vi "TDMS2TDMData.vi"(0 "tdms file in":refnum<k34>, 1 "Chunk Size":i64, 5 "group name":string, 9 "channel name":string, 11 "error in (no error)":errorcluster, 12 "Data type":i32, 13 "storage refnum":refnum<k20>) -> (4 "tdms file out":refnum<k34>, 6 "group name out":string, 15 "error out":errorcluster)   [LabVIEW 2017]
doc: "This VI transfers channel data from a TDMS channel to a TDM channel. The data is transfered in chunks of a certain size measured in samples until all the transfer is complete. If the TDMS channel contains a datatype not supported by the TDM storage format, then the data is coerced and the coercion is logged."
uses:
  <vilib>/Platform/storage/lvStorage.llb/_saveUInt8Channel.vi
  <vilib>/Utility/tdmsutil.llb/TDMS2TDMLogDataConversion.vi
  <vilib>/Platform/storage/lvStorage.llb/_saveInt16Channel.vi
  <vilib>/Platform/storage/lvStorage.llb/_saveInt32Channel.vi
  <vilib>/Platform/storage/lvStorage.llb/_saveFloat32Channel.vi
  <vilib>/Platform/storage/lvStorage.llb/_saveFloat64Channel.vi
  <vilib>/Platform/storage/lvStorage.llb/_saveStringChannel.vi
  <vilib>/Platform/storage/lvStorage.llb/_saveDateTimeChannel.vi
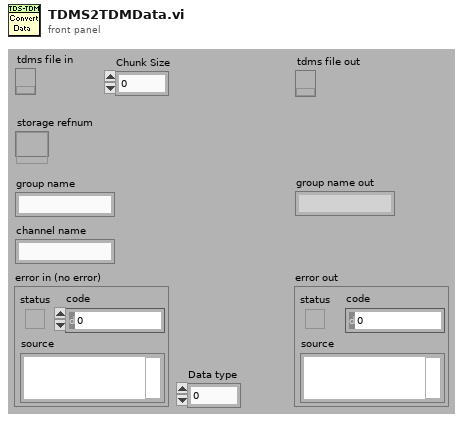
[diagram p1: front panel]
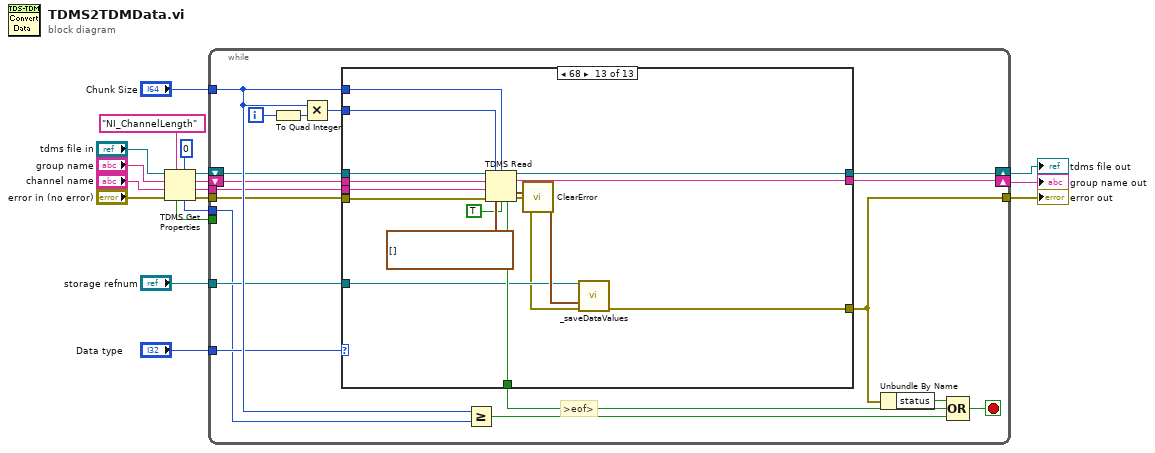
[diagram p0: block diagram]
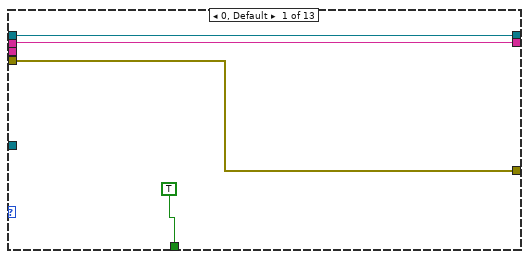
[diagram p2: hidden frame]
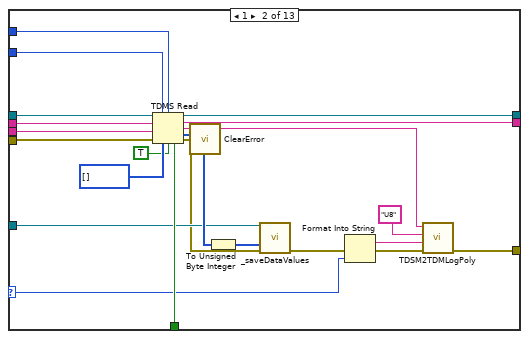
[diagram p3: hidden frame]
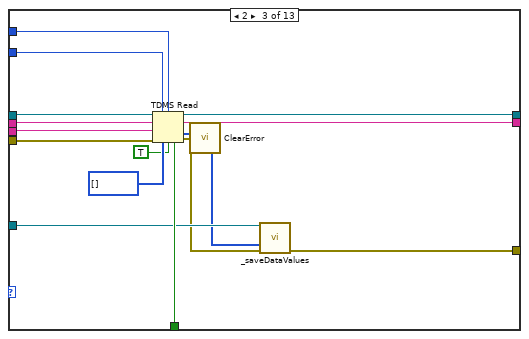
[diagram p4: hidden frame]
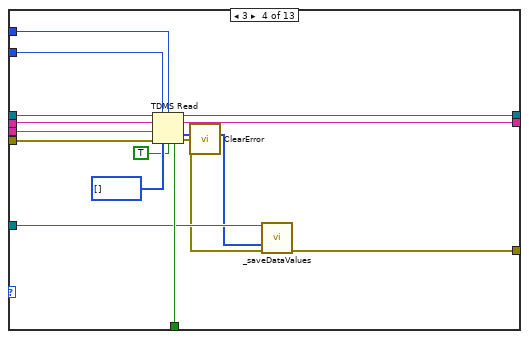
[diagram p5: hidden frame]
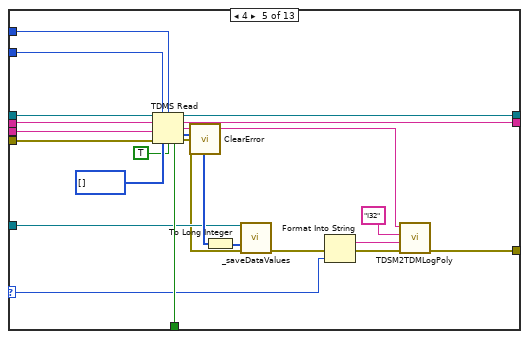
[diagram p6: hidden frame]
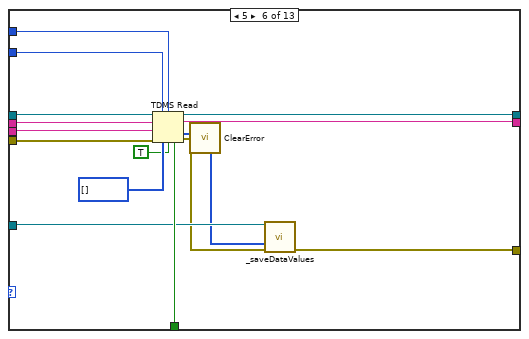
[diagram p7: hidden frame]
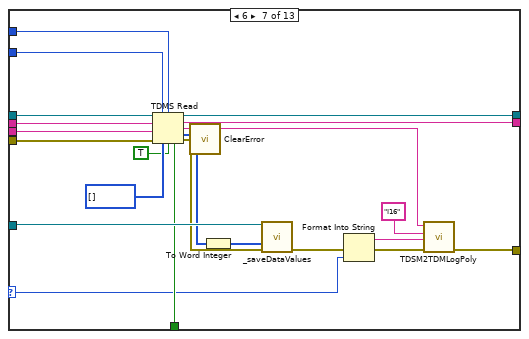
[diagram p8: hidden frame]
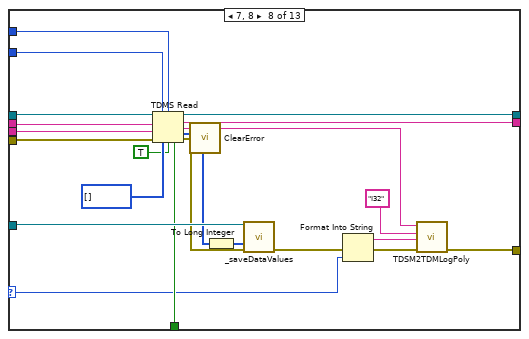
[diagram p9: hidden frame]
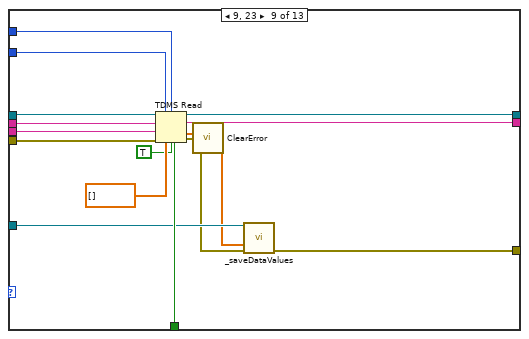
[diagram p10: hidden frame]
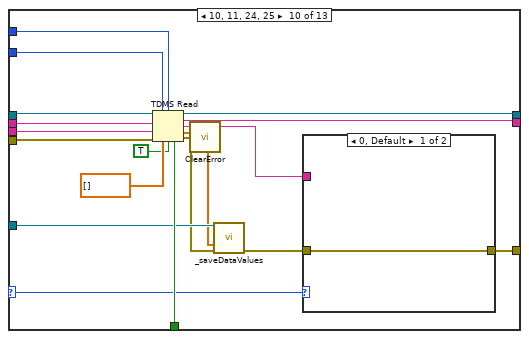
[diagram p11: hidden frame]
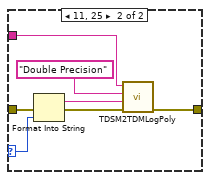
[diagram p12: hidden frame]
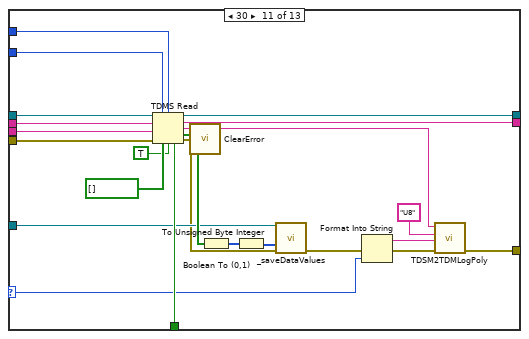
[diagram p13: hidden frame]
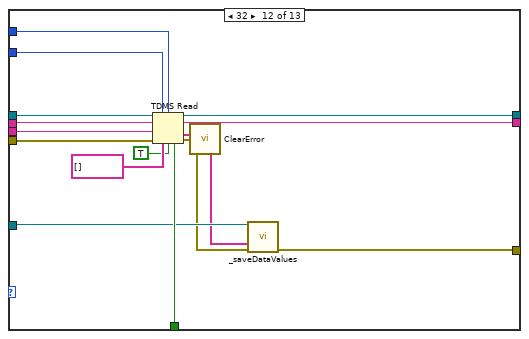
[diagram p14: hidden frame]
diagram:
  n1 = TDMS Get Properties(5:i64 0, 7:"NI_ChannelLength" ("property name"), 8:"error in (no error)", 9:"channel name", 10:"group name", 11:"tdms file in") -> (0:w5:errorcluster, 1:w6:string, 2:w7:string, 3:w8:refnum<k34>, 4:w3:i64, 6:w2:bool)
  n2 = while {
    tunnel: "storage refnum" -> [w34]
    tunnel: w6 -> [w31]
    tunnel: w5 -> [w30]
    shift-right: [w29] -> w15
    shift-left: w8 -> [w33]
    shift-right: [w28] -> w16
    shift-left: w7 -> [w32]
    tunnel: "Chunk Size" -> [w36]
    tunnel: [w35] -> w18
    tunnel: "Data type" -> [w24]
    tunnel: w3 -> [w21]
    tunnel: w2 -> [_]
    i -> [w27]
    stop <- w19 stop-if-true
    # ">eof>"
    n3 = To Quad Integer(1:w27) -> (0:w26:i64)
    n4 = Multiply(x=w36, y=w26) -> (x*y=w25:i64)
    n5 = case shown="68" w24 {
      selector: w24 -> [_ w46 _ _ w103 _ w142 w162 _ w202 w229 _ _]
      tunnel: w34 -> [_ w52 w68 w84 w107 w124 w157 w180 w185 w205 w236 w254 w269]
      tunnel: w33 -> [w40 w63 w79 w95 w118 w134 w156 w179 w196 w215 w247 w263 w279]
      tunnel: w32 -> [w39 w62 w78 w93 w117 w131 w154 w177 w194 w213 w244 w261 w278]
      tunnel: w31 -> [_ w61 w77 w92 w116 w130 w153 w176 w193 w212 w243 w256 w277]
      tunnel: w30 -> [w37 w60 w74 w91 w115 w128 w151 w178 w195 w211 w238 w260 w271]
      tunnel: [w40 w57 w76 w94 w113 w133 w155 w174 w192 w214 w246 w262 w276] -> w29
      tunnel: [w39 w56 w75 w89 w112 w129 w152 w173 w191 w206 w245 w255 w275] -> w28
      tunnel: w25 -> [_ w54 w71 w86 w110 w125 w148 w171 w188 w209 w240 w257 w273]
      tunnel: w36 -> [_ w55 w70 w87 w111 w126 w149 w172 w189 w210 w241 w258 w274]
      tunnel: [w37 w49 w69 w85 w101 w123 w139 w164 w186 w200 w230 w253 w268] -> w35
      tunnel: [TRUE ("eof") w53 w73 w90 w109 w132 w150 w175 w190 w208 w242 w259 w272] -> w22
      frame 0, Default {
      }
      frame 1 {
        n6 = TDMS Read(0:w63, 1:w54, 2:w55, 5:w62, 7:w61, 11:w60, 12:i8[] [], 13:TRUE ("return channels in file order? (F)")) -> (4:w57:refnum<k34>, 6:w56:string, 8:w43:string, 10:w59:i8[], 14:w53:bool, 15:w42:errorcluster)
        n7 = call <vilib>:"ClearError.vi"("error in (no error)"=w42) -> ("error out"=w50:errorcluster)
        n8 = To Unsigned Byte Integer(number=w59) -> (unsigned 8bit integer=w51:u8[])
        n9 = call-poly <vilib>:"_saveDataValues.vi"("Data object in"=w52, "Values"=w51, "error in (no error)"=w50) -> ("error out"=w48:errorcluster)  [unwired: 10 in, 2 out]
        n10 = Format Into String(error in=w48, w46) -> (resulting string=w45:string, error out=w47:errorcluster)  [unwired: 2 in]
        n11 = call-poly <vilib>:"TDSM2TDMLogPoly.vi"("error in (no error)"=w47, "Original Datatype"=w45, "New Datatype"="U8", "Channel Name"=w43) -> ("error out"=w49:errorcluster)  [unwired: 7 in]
      }
      frame 2 {
        n12 = TDMS Read(0:w79, 1:w71, 2:w70, 5:w78, 7:w77, 11:w74, 12:i16[] [], 13:TRUE ("return channels in file order? (F)")) -> (4:w76:refnum<k34>, 6:w75:string, 10:w67:i16[], 14:w73:bool, 15:w65:errorcluster)  [unwired: 1 out]
        n13 = call <vilib>:"ClearError.vi"("error in (no error)"=w65) -> ("error out"=w66:errorcluster)
        n14 = call-poly <vilib>:"_saveDataValues.vi"("Data object in"=w68, "Values"=w67, "error in (no error)"=w66) -> ("error out"=w69:errorcluster)  [unwired: 10 in, 2 out]
      }
      frame 3 {
        n15 = TDMS Read(0:w95, 1:w86, 2:w87, 5:w93, 7:w92, 11:w91, 12:i32[] [], 13:TRUE ("return channels in file order? (F)")) -> (4:w94:refnum<k34>, 6:w89:string, 10:w83:i32[], 14:w90:bool, 15:w81:errorcluster)  [unwired: 1 out]
        n16 = call <vilib>:"ClearError.vi"("error in (no error)"=w81) -> ("error out"=w82:errorcluster)
        n17 = call-poly <vilib>:"_saveDataValues.vi"("Data object in"=w84, "Values"=w83, "error in (no error)"=w82) -> ("error out"=w85:errorcluster)  [unwired: 10 in, 2 out]
      }
      frame 4 {
        n18 = TDMS Read(0:w118, 1:w110, 2:w111, 5:w117, 7:w116, 11:w115, 12:i64[] [], 13:TRUE ("return channels in file order? (F)")) -> (4:w113:refnum<k34>, 6:w112:string, 8:w98:string, 10:w108:i64[], 14:w109:bool, 15:w97:errorcluster)
        n19 = call <vilib>:"ClearError.vi"("error in (no error)"=w97) -> ("error out"=w105:errorcluster)
        n20 = To Long Integer(number=w108) -> (32bit integer=w106:i32[])
        n21 = call-poly <vilib>:"_saveDataValues.vi"("Data object in"=w107, "Values"=w106, "error in (no error)"=w105) -> ("error out"=w104:errorcluster)  [unwired: 10 in, 2 out]
        n22 = Format Into String(error in=w104, w103) -> (resulting string=w100:string, error out=w102:errorcluster)  [unwired: 2 in]
        n23 = call-poly <vilib>:"TDSM2TDMLogPoly.vi"("error in (no error)"=w102, "Original Datatype"=w100, "New Datatype"="I32", "Channel Name"=w98) -> ("error out"=w101:errorcluster)  [unwired: 7 in]
      }
      frame 5 {
        n24 = TDMS Read(0:w134, 1:w125, 2:w126, 5:w131, 7:w130, 11:w128, 12:u8[] [], 13:TRUE ("return channels in file order? (F)")) -> (4:w133:refnum<k34>, 6:w129:string, 10:w122:u8[], 14:w132:bool, 15:w120:errorcluster)  [unwired: 1 out]
        n25 = call <vilib>:"ClearError.vi"("error in (no error)"=w120) -> ("error out"=w121:errorcluster)
        n26 = call-poly <vilib>:"_saveDataValues.vi"("Data object in"=w124, "Values"=w122, "error in (no error)"=w121) -> ("error out"=w123:errorcluster)  [unwired: 10 in, 2 out]
      }
      frame 6 {
        n27 = TDMS Read(0:w156, 1:w148, 2:w149, 5:w154, 7:w153, 11:w151, 12:u16[] [], 13:TRUE ("return channels in file order? (F)")) -> (4:w155:refnum<k34>, 6:w152:string, 8:w137:string, 10:w146:u16[], 14:w150:bool, 15:w136:errorcluster)
        n28 = call <vilib>:"ClearError.vi"("error in (no error)"=w136) -> ("error out"=w144:errorcluster)
        n29 = To Word Integer(number=w146) -> (16bit integer=w145:i16[])
        n30 = call-poly <vilib>:"_saveDataValues.vi"("Data object in"=w157, "Values"=w145, "error in (no error)"=w144) -> ("error out"=w143:errorcluster)  [unwired: 10 in, 2 out]
        n31 = Format Into String(error in=w143, w142) -> (resulting string=w140:string, error out=w141:errorcluster)  [unwired: 2 in]
        n32 = call-poly <vilib>:"TDSM2TDMLogPoly.vi"("error in (no error)"=w141, "Original Datatype"=w140, "New Datatype"="I16", "Channel Name"=w137) -> ("error out"=w139:errorcluster)  [unwired: 7 in]
      }
      frame 7, 8 {
        n33 = TDMS Read(0:w179, 1:w171, 2:w172, 5:w177, 7:w176, 11:w178, 12:u32[] [], 13:TRUE ("return channels in file order? (F)")) -> (4:w174:refnum<k34>, 6:w173:string, 8:w160:string, 10:w169:u32[], 14:w175:bool, 15:w159:errorcluster)
        n34 = call <vilib>:"ClearError.vi"("error in (no error)"=w159) -> ("error out"=w167:errorcluster)
        n35 = To Long Integer(number=w169) -> (32bit integer=w168:i32[])
        n36 = call-poly <vilib>:"_saveDataValues.vi"("Data object in"=w180, "Values"=w168, "error in (no error)"=w167) -> ("error out"=w166:errorcluster)  [unwired: 10 in, 2 out]
        n37 = Format Into String(error in=w166, w162) -> (resulting string=w163:string, error out=w165:errorcluster)  [unwired: 2 in]
        n38 = call-poly <vilib>:"TDSM2TDMLogPoly.vi"("error in (no error)"=w165, "Original Datatype"=w163, "New Datatype"="I32", "Channel Name"=w160) -> ("error out"=w164:errorcluster)  [unwired: 7 in]
      }
      frame 9, 23 {
        n39 = TDMS Read(0:w196, 1:w188, 2:w189, 5:w194, 7:w193, 11:w195, 12:sgl[] [], 13:TRUE ("return channels in file order? (F)")) -> (4:w192:refnum<k34>, 6:w191:string, 10:w183:sgl[], 14:w190:bool, 15:w182:errorcluster)  [unwired: 1 out]
        n40 = call <vilib>:"ClearError.vi"("error in (no error)"=w182) -> ("error out"=w184:errorcluster)
        n41 = call-poly <vilib>:"_saveDataValues.vi"("Data object in"=w185, "Values"=w183, "error in (no error)"=w184) -> ("error out"=w186:errorcluster)  [unwired: 10 in, 2 out]
      }
      frame 10, 11, 24, 25 {
        n42 = TDMS Read(0:w215, 1:w209, 2:w210, 5:w213, 7:w212, 11:w211, 12:dbl[] [], 13:TRUE ("return channels in file order? (F)")) -> (4:w214:refnum<k34>, 6:w206:string, 8:w199:string, 10:w204:dbl[], 14:w208:bool, 15:w198:errorcluster)
        n43 = call <vilib>:"ClearError.vi"("error in (no error)"=w198) -> ("error out"=w203:errorcluster)
        n44 = call-poly <vilib>:"_saveDataValues.vi"("Data object in"=w205, "Values"=w204, "error in (no error)"=w203) -> ("error out"=w201:errorcluster)  [unwired: 10 in, 2 out]
        n45 = case shown="0, Default" w202 {
          selector: w202 -> [_ w222]
          tunnel: w201 -> [w216 w223]
          tunnel: [w216 w219] -> w200
          tunnel: w199 -> [_ w217]
          frame 0, Default {
          }
          frame 11, 25 {
            n46 = Format Into String(error in=w223, w222) -> (resulting string=w220:string, error out=w221:errorcluster)  [unwired: 2 in]
            n47 = call-poly <vilib>:"TDSM2TDMLogPoly.vi"("error in (no error)"=w221, "Original Datatype"=w220, "New Datatype"="Double Precision", "Channel Name"=w217) -> ("error out"=w219:errorcluster)  [unwired: 7 in]
          }
        }
      }
      frame 30 {
        n48 = TDMS Read(0:w247, 1:w240, 2:w241, 5:w244, 7:w243, 11:w238, 12:bool[] [], 13:TRUE ("return channels in file order? (F)")) -> (4:w246:refnum<k34>, 6:w245:string, 8:w226:string, 10:w237:bool[], 14:w242:bool, 15:w225:errorcluster)
        n49 = call <vilib>:"ClearError.vi"("error in (no error)"=w225) -> ("error out"=w235:errorcluster)
        n50 = Boolean To (0,1)(Boolean=w237) -> (0, 1=w234:i16[])
        n51 = To Unsigned Byte Integer(number=w234) -> (unsigned 8bit integer=w233:u8[])
        n52 = call-poly <vilib>:"_saveDataValues.vi"("Data object in"=w236, "Values"=w233, "error in (no error)"=w235) -> ("error out"=w232:errorcluster)  [unwired: 10 in, 2 out]
        n53 = Format Into String(error in=w232, w229) -> (resulting string=w228:string, error out=w231:errorcluster)  [unwired: 2 in]
        n54 = call-poly <vilib>:"TDSM2TDMLogPoly.vi"("error in (no error)"=w231, "Original Datatype"=w228, "New Datatype"="U8", "Channel Name"=w226) -> ("error out"=w230:errorcluster)  [unwired: 7 in]
      }
      frame 32 {
        n55 = TDMS Read(0:w263, 1:w257, 2:w258, 5:w261, 7:w256, 11:w260, 12:string[] [], 13:TRUE ("return channels in file order? (F)")) -> (4:w262:refnum<k34>, 6:w255:string, 10:w251:string[], 14:w259:bool, 15:w249:errorcluster)  [unwired: 1 out]
        n56 = call <vilib>:"ClearError.vi"("error in (no error)"=w249) -> ("error out"=w252:errorcluster)
        n57 = call-poly <vilib>:"_saveDataValues.vi"("Data object in"=w254, "Values"=w251, "error in (no error)"=w252) -> ("error out"=w253:errorcluster)  [unwired: 10 in, 2 out]
      }
      frame 68 {
        n58 = TDMS Read(0:w279, 1:w273, 2:w274, 5:w278, 7:w277, 11:w271, 12:timestamp[] [], 13:TRUE ("return channels in file order? (F)")) -> (4:w276:refnum<k34>, 6:w275:string, 10:w270:timestamp[], 14:w272:bool, 15:w265:errorcluster)  [unwired: 1 out]
        n59 = call <vilib>:"ClearError.vi"("error in (no error)"=w265) -> ("error out"=w266:errorcluster)
        n60 = call-poly <vilib>:"_saveDataValues.vi"("Data object in"=w269, "Values"=w270, "error in (no error)"=w266) -> ("error out"=w268:errorcluster)  [unwired: 10 in, 2 out]
      }
    }
    n61 = Greater Or Equal?(x=w36, y=w21) -> (x >= y?=w20:bool)
    n62 = Unbundle By Name(w35) -> ("status"=w23:bool)
    n63 = Compound Arithmetic op=OR(w23, w22, w20) -> (w19:bool)
  }
  "error out" <- w18
  "group name out" <- w16
  "tdms file out" <- w15
